vi "Open Debug Process.vi"(8 "error in (no error)":errorcluster, 11 "DebuggingTerminal in":refnum<class "DebuggingTerminal.lvclass">) -> (0 "error out":errorcluster, 3 "DebuggingTerminal out":refnum<class "DebuggingTerminal.lvclass">)   [LabVIEW 2013, in "MQTT Base.lvlib" / "DebuggingTerminal.lvclass"]
uses:
  DebuggingTerminal.lvclass
  Process.vi
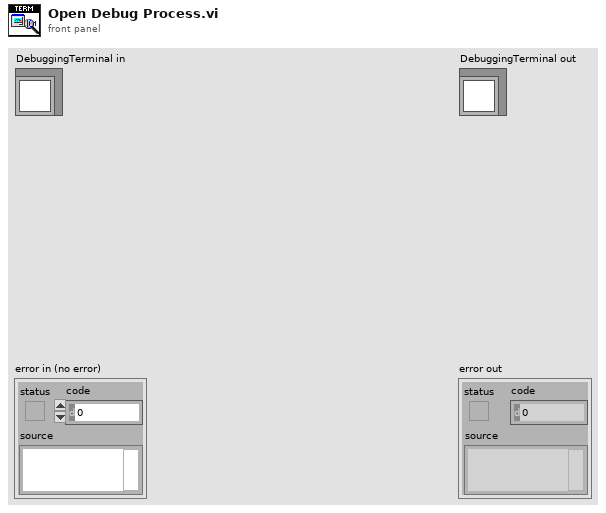
[diagram p1: front panel]
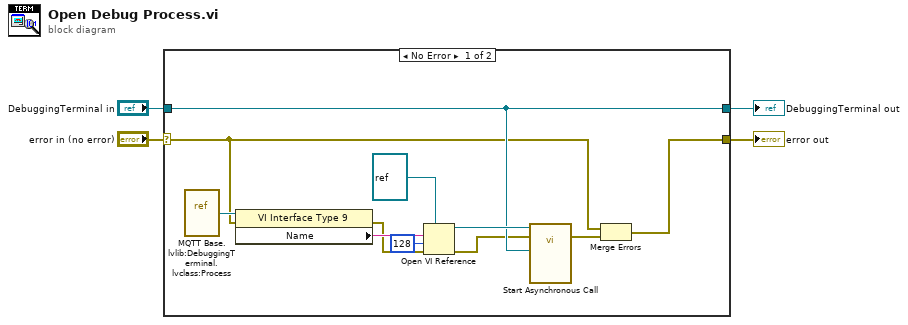
[diagram p0: block diagram]
diagram:
  n1 = case shown="No Error" "error in (no error)" {
    selector: "error in (no error)" -> [w8 w17]
    tunnel: [w7 w17] -> w3
    tunnel: [w13 w16] -> w1
    tunnel: "DebuggingTerminal in" -> [w13 w16]
    frame No Error {
      n2 = vi-ref "MQTT Base.lvlib:DebuggingTerminal.lvclass:Process.vi"() -> (w12:refnum<vi>)
      n3 = property class="VI Interface Type 9"(reference=w12, error in=w8) -> (error out=w10:errorcluster, "Name"=w11:string)  [unwired: 1 out]
      n4 = Open VI Reference(type specifier VI Refnum (for type only)=refnum<vi> refnum, vi path=w11, options=128, error in (no error)=w10) -> (vi reference=w15:refnum<vi>, error out=w5:errorcluster)  [unwired: 2 in]
      n5 = call-by-ref "Start Asynchronous Call"(reference=w15, error in=w5, "DebuggingTerminal"=w13) -> (error out=w9:errorcluster)  [unwired: 11 in, 1 out]
      n6 = Merge Errors(w8, w9) -> (w7:errorcluster)
    }
    frame Error {
    }
  }
  "error out" <- w3
  "DebuggingTerminal out" <- w1
